vi "Test Method 1.vi"(8 "error in (no error)":errorcluster, 11 "Test Case In":refnum<class "Global Fixture Demo Test Case.lvclass">) -> (0 "error out":errorcluster, 3 "Test Case Out":refnum<class "Global Fixture Demo Test Case.lvclass">)   [LabVIEW 2020, in "Global Fixture Demo Test Case.lvclass"]
uses:
  Global Fixture Demo Test Case.lvclass
  C:/Program Files (x86)/National Instruments/LabVIEW 2020/vi.lib/Astemes/LUnit/Test Case.lvclass
  <vilib>/Astemes/LUnit/Test Case.lvclass/Test Case.ctl
  4993e8ee-a06a-463a-9684-69129f64d5ce.vi
  <vilib>/Astemes/LUnit/Append Pass Result.vi
  <vilib>/Astemes/LUnit/Append Fail Result.vi
  <vilib>/Astemes/LUnit/Describe Comparison.vi
  <vilib>/Astemes/LUnit/Compare Variants.vi
  <vilib>/Astemes/LUnit/Run In UI.vi
  <vilib>/Utility/error.llb/Clear Errors.vi
  <vilib>/Astemes/LUnit/Describe Variant.vi
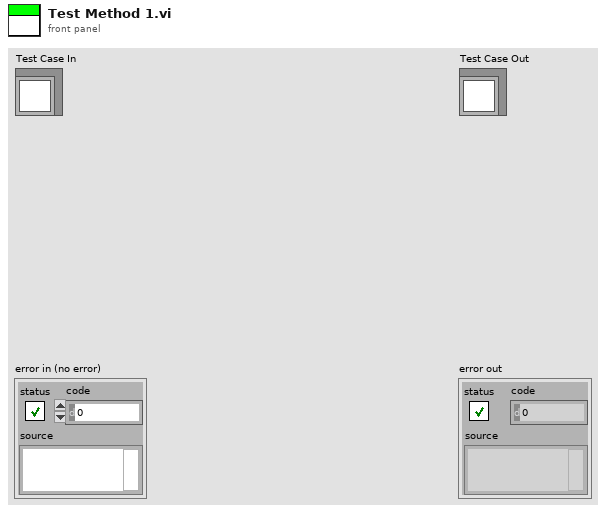
[diagram p1: front panel]
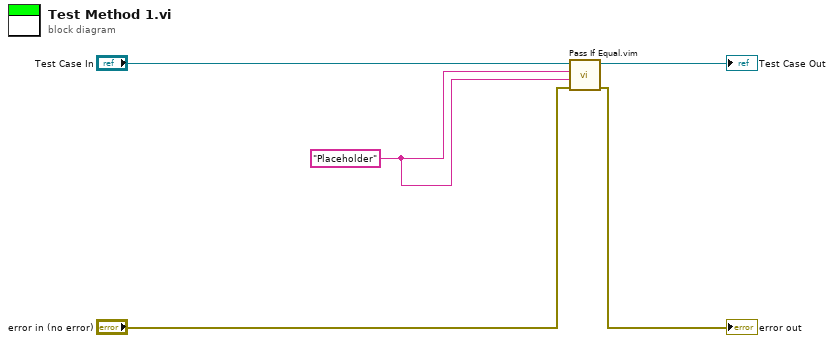
[diagram p0: block diagram]
diagram:
  w1 = "Placeholder"
  n1 = call "Pass If Equal.vim"("error in (no error)"="error in (no error)", "Actual"=w1, "Expected"=w1, "LUnit Test Case In"="Test Case In") -> ("error out"=→"error out":errorcluster, "LUnit Test Case Out"=→"Test Case Out":refnum<class "Global Fixture Demo Test Case.lvclass">)  [unwired: 6 in]
